vi "ApostrapheDBHandler.vi"(1 "string in":string) -> (0 "string out":string)   [LabVIEW 2024]
uses:
  <vilib>/Utility/error.llb/Trim Whitespace One-Sided.vi
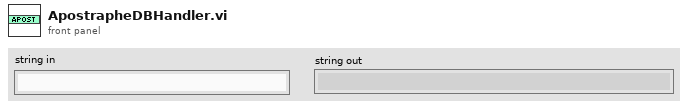
[diagram p1: front panel]
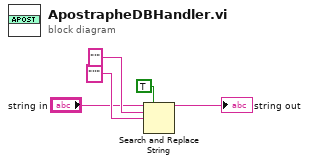
[diagram p0: block diagram]
diagram:
  n1 = Search and Replace String(replace all?=TRUE ("replace all? (F)"), input string="string in", search string="'", replace string="''" ("search string")) -> (result string=→"string out":string)  [unwired: 4 in, 3 out]
